vi "test device name mismatch error.vi"(8 "error in (no error)":errorcluster, 11 "TestCase in":refnum<class "PharLap System Tests.lvclass">) -> (0 "error out":errorcluster, 3 "TestCase out":refnum<class "PharLap System Tests.lvclass">)   [LabVIEW 2015, in "PharLap System Tests.lvclass"]
uses:
  PharLap System Tests.lvclass
  <vilib>/addons/_JKI Toolkits/VI Tester/TestCase.llb/TestCase.lvclass
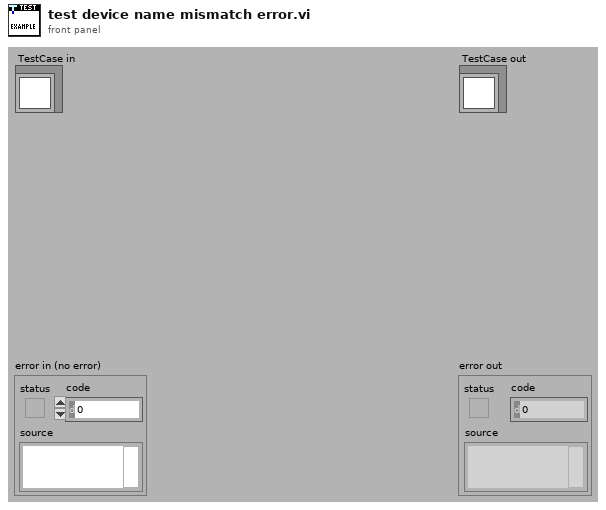
[diagram p1: front panel]
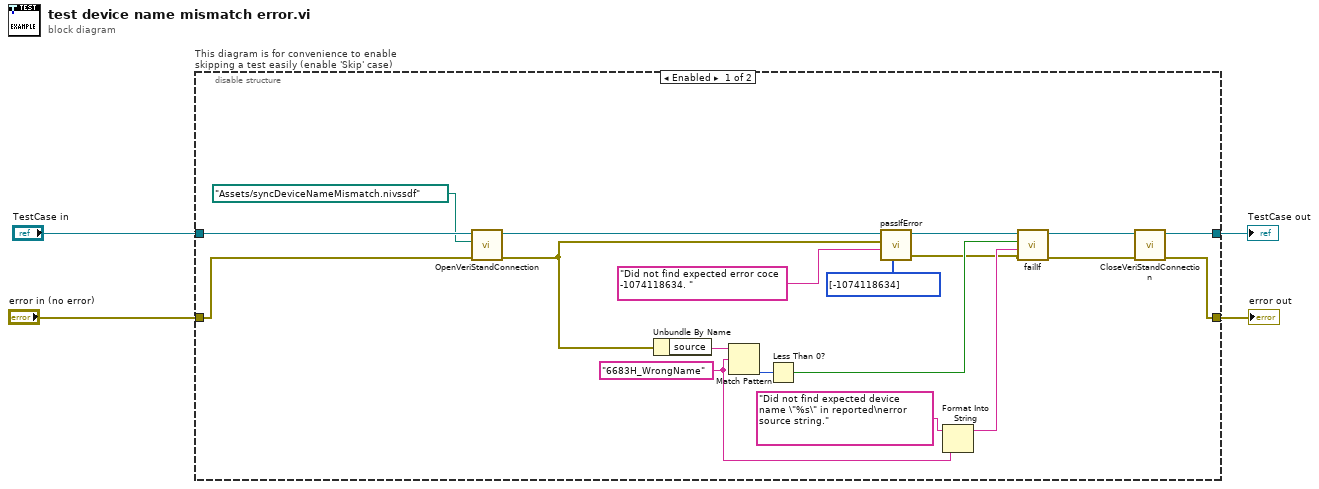
[diagram p0: block diagram]
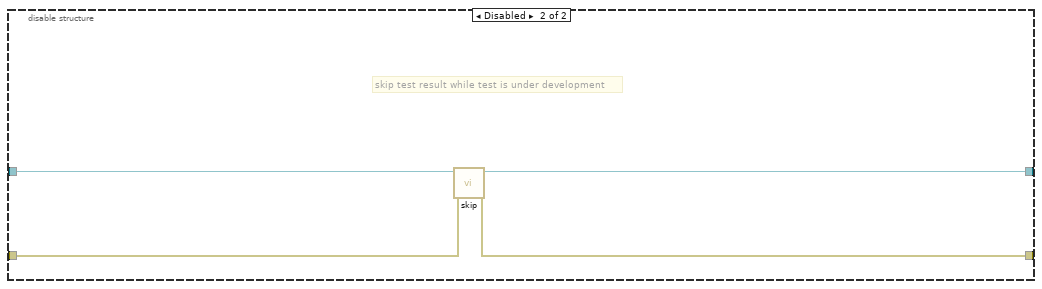
[diagram p2: hidden frame]
diagram:
  n1 = disable-structure "This diagram is for convenience to enable skipping a test easily (enable 'Skip' case)" shown="Enabled" {
    disable-tunnel: "TestCase in" -> [w23 w27]
    disable-tunnel: [w15 w25] -> w1
    disable-tunnel: [w14 w26] -> w3
    disable-tunnel: "error in (no error)" -> [w22 w24]
    frame Enabled {
      w17 = "6683H_WrongName" ("regular expression")
      n2 = call-dynamic "OpenVeriStandConnection.vi"("error in (no error)"=w22, "System Definition File"=path "Assets/syncDeviceNameMismatch.nivssdf", "VeriStand Test Case in"=w23) -> ("error out"=w5:errorcluster, "VeriStand Test Case out"=w20:refnum<class "PharLap System Tests.lvclass">)  [unwired: 7 in]
      n3 = Unbundle By Name(w5) -> ("source"=w18:string)
      n4 = Match Pattern(string=w18, regular expression=w17) -> (offset past match=w9:i32)  [unwired: 1 in, 3 out]
      n5 = Less Than 0?(x=w9) -> (x < 0?=w8:bool)
      n6 = call-dynamic "passIfError.vi"("passing error codes (default = any error code)"=i32[] [-1074118634], "task (\"\")"="Did not find expected error coce -1074118634. ", "error"=w5, "TestCase in"=w20) -> ("error out"=w6:errorcluster, "TestCase out"=w12:refnum<class "PharLap System Tests.lvclass">)  [unwired: 6 in]
      n7 = Format Into String(format string="Did not find expected device name \"%s\" in reported\nerror source string.", w17) -> (resulting string=w10:string)  [unwired: 2 in, 1 out]
      n8 = call-dynamic "failIf.vi"("error in (no error)"=w6, "message (\"\")"=w10, "fail"=w8, "TestCase in"=w12) -> ("error out"=w7:errorcluster, "TestCase out"=w11:refnum<class "PharLap System Tests.lvclass">)  [unwired: 6 in]
      n9 = call-dynamic "CloseVeriStandConnection.vi"("error in (no error)"=w7, "VeriStand Test Case in"=w11) -> ("error out"=w14:errorcluster, "VeriStand Test Case out"=w15:refnum<class "PharLap System Tests.lvclass">)  [unwired: 8 in]
    }
    frame Disabled {
      # "skip test result while test is under development"
      n10 = call <vilib>:"skip.vi"("error in (no error)"=w24, "TestCase in"=w27) -> ("error out"=w26:errorcluster, "TestCase out"=w25:refnum<class "PharLap System Tests.lvclass">)  [unwired: 8 in]
    }
  }
  "error out" <- w3
  "TestCase out" <- w1
